vi "InimigoMaisPerigoso.vi"(4 "Raio Gol Area":dbl format="%#_13g", 5 "Field Length":dbl format="%#_13g", 6 "Y Center Back":dbl format="%#_13g", 7 "X Center Back":dbl format="%#_13g", 8 "Y bola":dbl format="%#_13g", 9 "X bola":dbl format="%#_13g", 10 "Y inimigo":dbl format="%#_13g", 11 "X inimgo":dbl format="%#_13g") -> (3 "Fator de Perigo":dbl format="%#_13g")   [LabVIEW 2017]
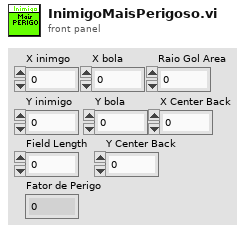
[diagram p1: front panel]
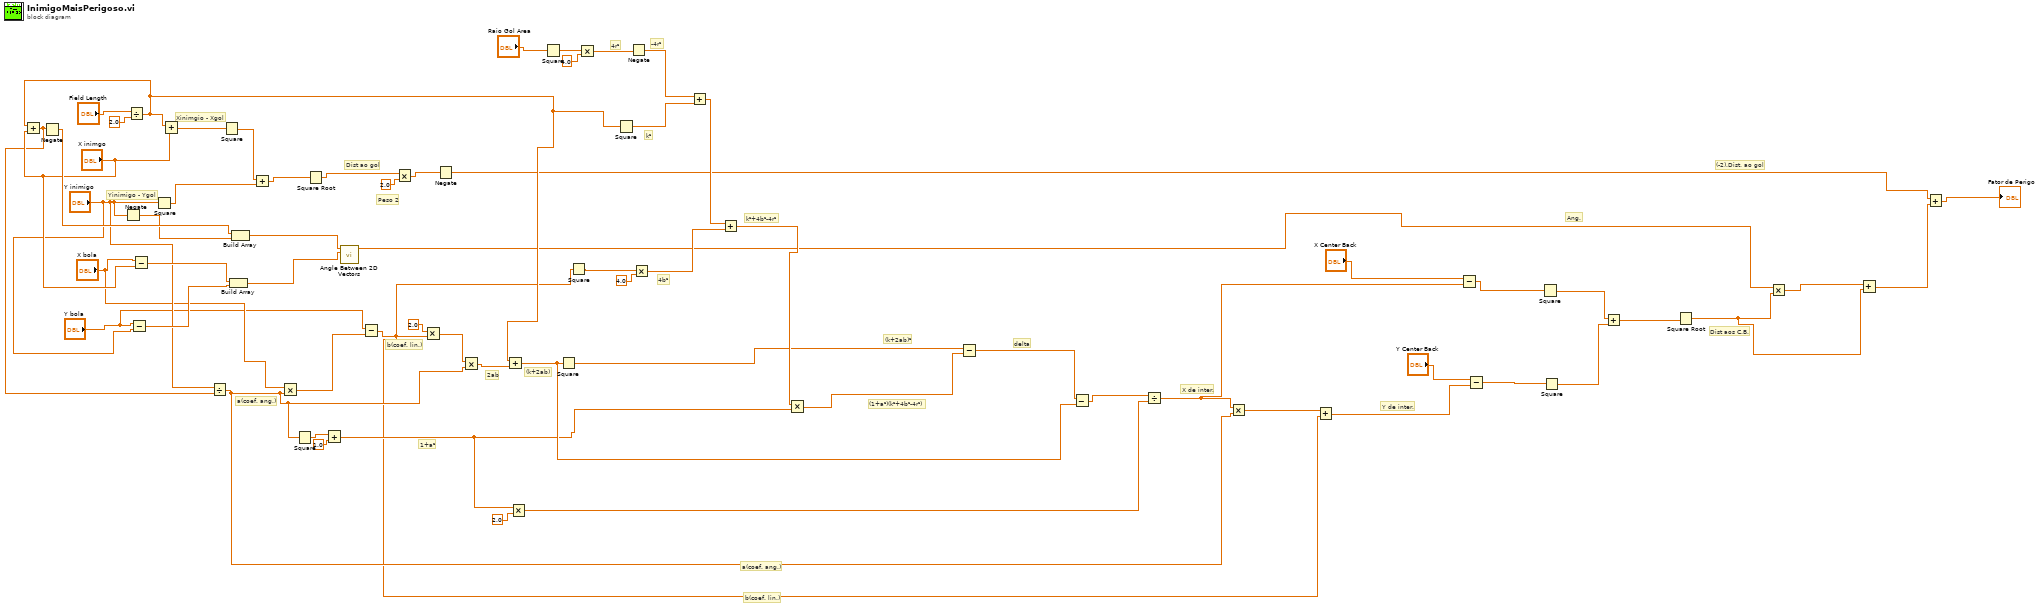
[diagram p0: block diagram]
diagram:
  # "(-2).Dist. ao gol"
  # "Ang."
  # "Dist aos C.B."
  # "Y de inter."
  # "b(coef. lin.)"
  # "a(coef. ang.)"
  # "X de inter."
  # "delta"
  # "(1+a²)(k²+4b²-4r²)"
  # "(k+2ab)²"
  # "k²+4b²-4r²"
  # "-4r²"
  # "4b²"
  # "4r²"
  # "k²"
  # "1+a²"
  # "(k+2ab)"
  # "2ab"
  # "b(coef. lin.)"
  # "a(coef. ang.)"
  # "Peso 2"
  # "Dist ao gol"
  # "Yinimigo - Ygol"
  # "Xinimgio - Xgol"
  n1 = Negate(x="Y inimigo") -> (-x=w54:dbl)
  n2 = Divide(x="Field Length", y=2.0 ("x")) -> (x/y=w34:dbl)
  n3 = Add(x=w34, y="X inimgo") -> (x+y=w47:dbl)
  n4 = Negate(x=w47) -> (-x=w55:dbl)
  n5 = Subtract(x="Y bola", y="Y inimigo") -> (x-y=w49:dbl)
  n6 = Subtract(x="X bola", y="X inimgo") -> (x-y=w50:dbl)
  n7 = Square(x="Y inimigo") -> (x^2=w62:dbl)
  n8 = Add(x=w34, y="X inimgo") -> (x+y=w63:dbl)
  n9 = Divide(x="Y inimigo", y=w47) -> (x/y=w18:dbl)
  n10 = Square(x=w63) -> (x^2=w61:dbl)
  n11 = Build Array(w50, w49) -> (w52:dbl[])
  n12 = Build Array(w55, w54) -> (w53:dbl[])
  n13 = Add(x=w61, y=w62) -> (x+y=w60:dbl)
  n14 = Multiply(x="X bola", y=w18) -> (x*y=w45:dbl)
  n15 = Square(x=w18) -> (x^2=w37:dbl)
  n16 = Square Root(x=w60) -> (sqrt(x)=w59:dbl)
  n17 = Add(x=w37, y=1.0) -> (x+y=w21:dbl)
  n18 = call "Angle Between 2D Vectors.vi"("Array"=w52, "Array 2"=w53) -> ("Numeric"=w6:dbl)  [unwired: 9 in]
  n19 = Subtract(x="Y bola", y=w45) -> (x-y=w16:dbl)
  n20 = Multiply(x=w59, y=2.0) -> (x*y=w57:dbl)
  n21 = Multiply(x=2.0, y=w16) -> (x*y=w39:dbl)
  n22 = Negate(x=w57) -> (-x=w2:dbl)
  n23 = Multiply(x=w39, y=w18) -> (x*y=w38:dbl)
  n24 = Add(x=w34, y=w38) -> (x+y=w23:dbl)
  n25 = Multiply(x=w21, y=2.0) -> (x*y=w19:dbl)
  n26 = Square(x="Raio Gol Area") -> (x^2=w42:dbl)
  n27 = Square(x=w23) -> (x^2=w26:dbl)
  n28 = Square(x=w16) -> (x^2=w30:dbl)
  n29 = Multiply(x=w42, y=4.0) -> (x*y=w35:dbl)
  n30 = Square(x=w34) -> (x^2=w32:dbl)
  n31 = Negate(x=w35) -> (-x=w33:dbl)
  n32 = Multiply(x=w30, y=4.0) -> (x*y=w29:dbl)
  n33 = Add(x=w33, y=w32) -> (x+y=w28:dbl)
  n34 = Add(x=w28, y=w29) -> (x+y=w27:dbl)
  n35 = Multiply(x=w27, y=w21) -> (x*y=w25:dbl)
  n36 = Subtract(x=w26, y=w25) -> (x-y=w24:dbl)
  n37 = Subtract(x=w24, y=w23) -> (x-y=w22:dbl)
  n38 = Divide(x=w22, y=w19) -> (x/y=w12:dbl)
  n39 = Multiply(x=w12, y=w18) -> (x*y=w17:dbl)
  n40 = Add(x=w17, y=w16) -> (x+y=w14:dbl)
  n41 = Subtract(x="X Center Back", y=w12) -> (x-y=w11:dbl)
  n42 = Subtract(x="Y Center Back", y=w14) -> (x-y=w10:dbl)
  n43 = Square(x=w11) -> (x^2=w9:dbl)
  n44 = Square(x=w10) -> (x^2=w8:dbl)
  n45 = Add(x=w9, y=w8) -> (x+y=w7:dbl)
  n46 = Square Root(x=w7) -> (sqrt(x)=w5:dbl)
  n47 = Multiply(x=w6, y=w5) -> (x*y=w4:dbl)
  n48 = Add(x=w4, y=w5) -> (x+y=w3:dbl)
  n49 = Add(x=w2, y=w3) -> (x+y=→"Fator de Perigo":dbl)
